vi "执行次数子VI1.vi"(1 "执行次数":i32) -> (0 "HEX显示":string)   [LabVIEW 2014]
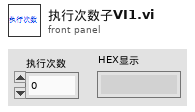
[diagram p1: front panel]
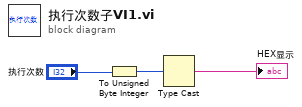
[diagram p0: block diagram]
diagram:
  n1 = To Unsigned Byte Integer(number="执行次数") -> (unsigned 8bit integer=w2:u8)
  n2 = Type Cast(x=w2) -> (*(type *) &x=→"HEX显示":string)  [unwired: 1 in]
